vi "Teleop.vi"(10 "Match Info":T1={"Autonomous Elapsed Seconds"=0.0, "TeleOp Elapsed Seconds"=0.0, "Disabled Elapsed Seconds"=0.0, "Visited Autonomous"=FALSE, "Visited TeleOp"=FALSE, "Visited Disabled"=FALSE, "Autonomous Settings"={"Autonomous Style"=enum."Independent", "VI Refnum"=refnum}}, 11 "Call Context":T2) -> ()   [LabVIEW 2018]
doc: "This VI is called for each TeleOp packet received from the DS where the robot is not disabled. It is often used to read from the joysticks and update I/O or to update setpoints for timed control loops. It should complete and return within 20 milliseconds or it may miss DS packets."
uses:
  <vilib>/Rock Robotics/Network Tables/NT Write Numeric Array.vi
  <vilib>/Rock Robotics/Network Tables/NT Read Boolean.vi
  <vilib>/Rock Robotics/Network Tables/NT Write Boolean Array.vi
  <vilib>/Rock Robotics/Network Tables/NT Read Number.vi
  <vilib>/Rock Robotics/Network Tables/NT Write Number.vi
  <vilib>/Rock Robotics/WPI/DriverStation/WPI_DriverStationMatch Info.ctl
  <vilib>/Rock Robotics/WPI/DriverStation/WPI_DriverStationDerivedRobotMode.ctl
panel:
  out "Color":u32(colorbox)
  out "Measured Color":cluster{"R":dbl, "G":dbl, "B":dbl}
  out "Sample Slider 0":dbl(slide) scale=0.0..5.0
  out "Sample Boolean 1":bool
  out "Sample Boolean 0":bool
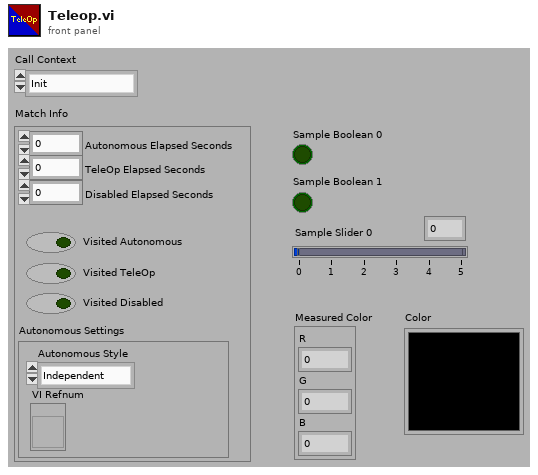
[diagram p1: front panel]
types:
  T1 = typedef "WPI_DriverStationMatch Info.ctl" = cluster{"Autonomous Elapsed Seconds":dbl, "TeleOp Elapsed Seconds":dbl, "Disabled Elapsed Seconds":dbl, "Visited Autonomous":bool, "Visited TeleOp":bool, "Visited Disabled":bool, "Autonomous Settings":cluster{"Autonomous Style":enum16{"Iterative", "Independent"}, "VI Refnum":refnum<vi>}}
  T2 = typedef "WPI_DriverStationDerivedRobotMode.ctl" = enum16{"Init", "Execute", "Stop"}
  T3 = typedef "WPI_RobotDriveDevRef.ctl" = cluster{"DevStatus":errorcluster, "Motors[]":T4[], "Square Inputs":bool, "Max Output":dbl}
  T4 = typedef "WPI_MotorControlDeviceRef.ctl" = cluster{"DeviceStatus":errorcluster, "Type":T5, "PWM":cluster{"PWM Channel":T6, "DeadBand":T7}, "CAN":cluster{"Device Number":u8, "SetOutput VI Ref":variant, "GetOutput VI Ref":variant, "Enable VI Ref":variant, "Disable VI Ref":variant, "Data":variant}, "Invert":bool, "DIO PWM":cluster{"PWM \"Enable\" Channel":T6, "DIOChannel":T8, "PWM Rate":dbl}}
  T5 = typedef "WPI_MotorControlType.ctl" = enum16{"PWM", "CAN", "DIO PWM"}
  T6 = typedef "FPGA_DIOPWMChannel.ctl" = enum8{"PWM 0", "PWM 1", "PWM 2", "PWM 3", "PWM 4", "PWM 5", "PWM 6", "PWM 7", "PWM 8", "PWM 9", "PWM MXP 0", "PWM MXP 1", "PWM MXP 2", "PWM MXP 3", "PWM MXP 4", "PWM MXP 5", "PWM MXP 6", "PWM MXP 7", "PWM MXP 8", "PWM MXP 9", "Invalid"}
  T7 = typedef "WPI_PWMDeadband.ctl" = cluster{"Name":string, "maxPositivePwm":i32, "minPositivePwm":i32, "centerPwm":i32, "maxNegativePwm":i32, "minNegativePwm":i32, "angularRange":u16}
  T8 = typedef "FPGA_DIOChannel.ctl" = enum8{"DIO 0", "DIO 1", "DIO 2", "DIO 3", "DIO 4", "DIO 5", "DIO 6", "DIO 7", "DIO 8", "DIO 9", "DIO MXP 0", "DIO MXP 1", "DIO MXP 2", "DIO MXP 3", "DIO MXP 4", "DIO MXP 5", "DIO MXP 6", "DIO MXP 7", "DIO MXP 8", "DIO MXP 9", "DIO MXP 10", "DIO MXP 11", "DIO MXP 12", "DIO MXP 13", "DIO MXP 14", "DIO MXP 15", "SPI Port CS1", "SPI Port CS2", "SPI Port CS3", "SPI Port MISO", "SPI Port MOSI", "Invalid"}
  T9 = typedef "WPI_JoystickDevRef.ctl" = cluster{"Device":T10}
  T10 = typedef "WPI_JoystickDeviceEnum.ctl" = enum16{"USB 0", "USB 1", "USB 2", "USB 3", "USB 4", "USB 5"}
  T11 = typedef "Color Sensor V3 DevRef.ctl" = cluster{"I2CDevRef":T12}
  T12 = typedef "WPI_I2CDevRef.ctl" = cluster{"DevStatus":errorcluster, "Device Address":u8, "Handle":i32, "I2C Bus":T13}
  T13 = typedef "i2c_bus.ctl" = enum16{"I2C On-Board", "I2C MXP", "Invalid"}
  T14 = typedef "WPI_GyroDevRef.ctl" = cluster{"DevStatus":errorcluster, "Analog Channel":T15, "Gain (VoltsPerDegree/Second)":dbl, "Gyro Type":enum16{"Analog", "XRS450"}, "Handle":i32, "SPI Bus":T16, "Device Found":bool, "Sample Rate":dbl, "Calibrate On Open":bool, "Offset":dbl}
  T15 = typedef "FPGA_AIChannel.ctl" = enum8{"AI 0", "AI 1", "AI 2", "AI 3", "AI MXP 0", "AI MXP 1", "AI MXP 2", "AI MXP 3", "Invalid"}
  T16 = typedef "spi_bus.ctl" = enum16{"SPI On-Board, CS0", "SPI On-Board, CS1", "SPI On-Board, CS2", "SPI On-Board, CS3", "SPI MXP", "Invalid"}
  T17 = typedef "WPI_CompressorDevRef.ctl" = cluster{"DevStatus":errorcluster, "Pneumatics Control Module":u8}
  T18 = typedef "WPI_EncoderDevRef.ctl" = cluster{"DevStatus":errorcluster, "EncoderIndex":T19, "CounterIndex":T20, "DistancePerCount":dbl, "Decoding Type":T21}
  T19 = typedef "FPGA_EncoderIdx.ctl" = enum8{"Enc 0", "Enc 1", "Enc 2", "Enc 3", "Enc 4", "Enc 5", "Enc 6", "Enc 7", "Invalid"}
  T20 = typedef "FPGA_CounterCtrSystemIndex.ctl" = enum8{"Ctr 0", "Ctr 1", "Ctr 2", "Ctr 3", "Ctr 4", "Ctr 5", "Ctr 6", "Ctr 7", "Invalid"}
  T21 = typedef "WPI_EncoderType.ctl" = enum16{"1x", "2x", "4x"}
  T22 = typedef "WPI_AnalogChannelDevRef.ctl" = cluster{"DevStatus":errorcluster, "Analog Channel":T15}
  T23 = typedef "WPI_AccelerometerDevRef.ctl" = cluster{"DevStatus":errorcluster, "Scaling":T24, "Analog Channels":T25, "I2C Bus":T13, "SPI Bus":T16, "Accel Range":T26, "ADXL Axes":T27, "Handle":i32, "Device Address":u8, "Accel Type":enum16{"Analog", "ADXL345 I2C", "ADXL345 SPI", "Internal", "ADXL362 SPI"}}
  T24 = typedef "WPI_AccelerometerScaling.ctl" = cluster{"Gain (VoltsPerG)":dbl, "Center Voltage":dbl}
  T25 = typedef "WPI_AccelerometerAnalogChannels.ctl" = cluster{"X-Axis":T15, "Y-Axis":T15, "Z-Axis":T15}
  T26 = typedef "ADXL345 Range.ctl" = u8
  T27 = typedef "WPI_AccelerometerADXL345 Axes.ctl" = cluster{"X-Axis":bool, "Y-Axis":bool, "Z-Axis":bool}
  T28 = cluster{"X-Axis":dbl, "Y-Axis":dbl, "Z-Axis":dbl}
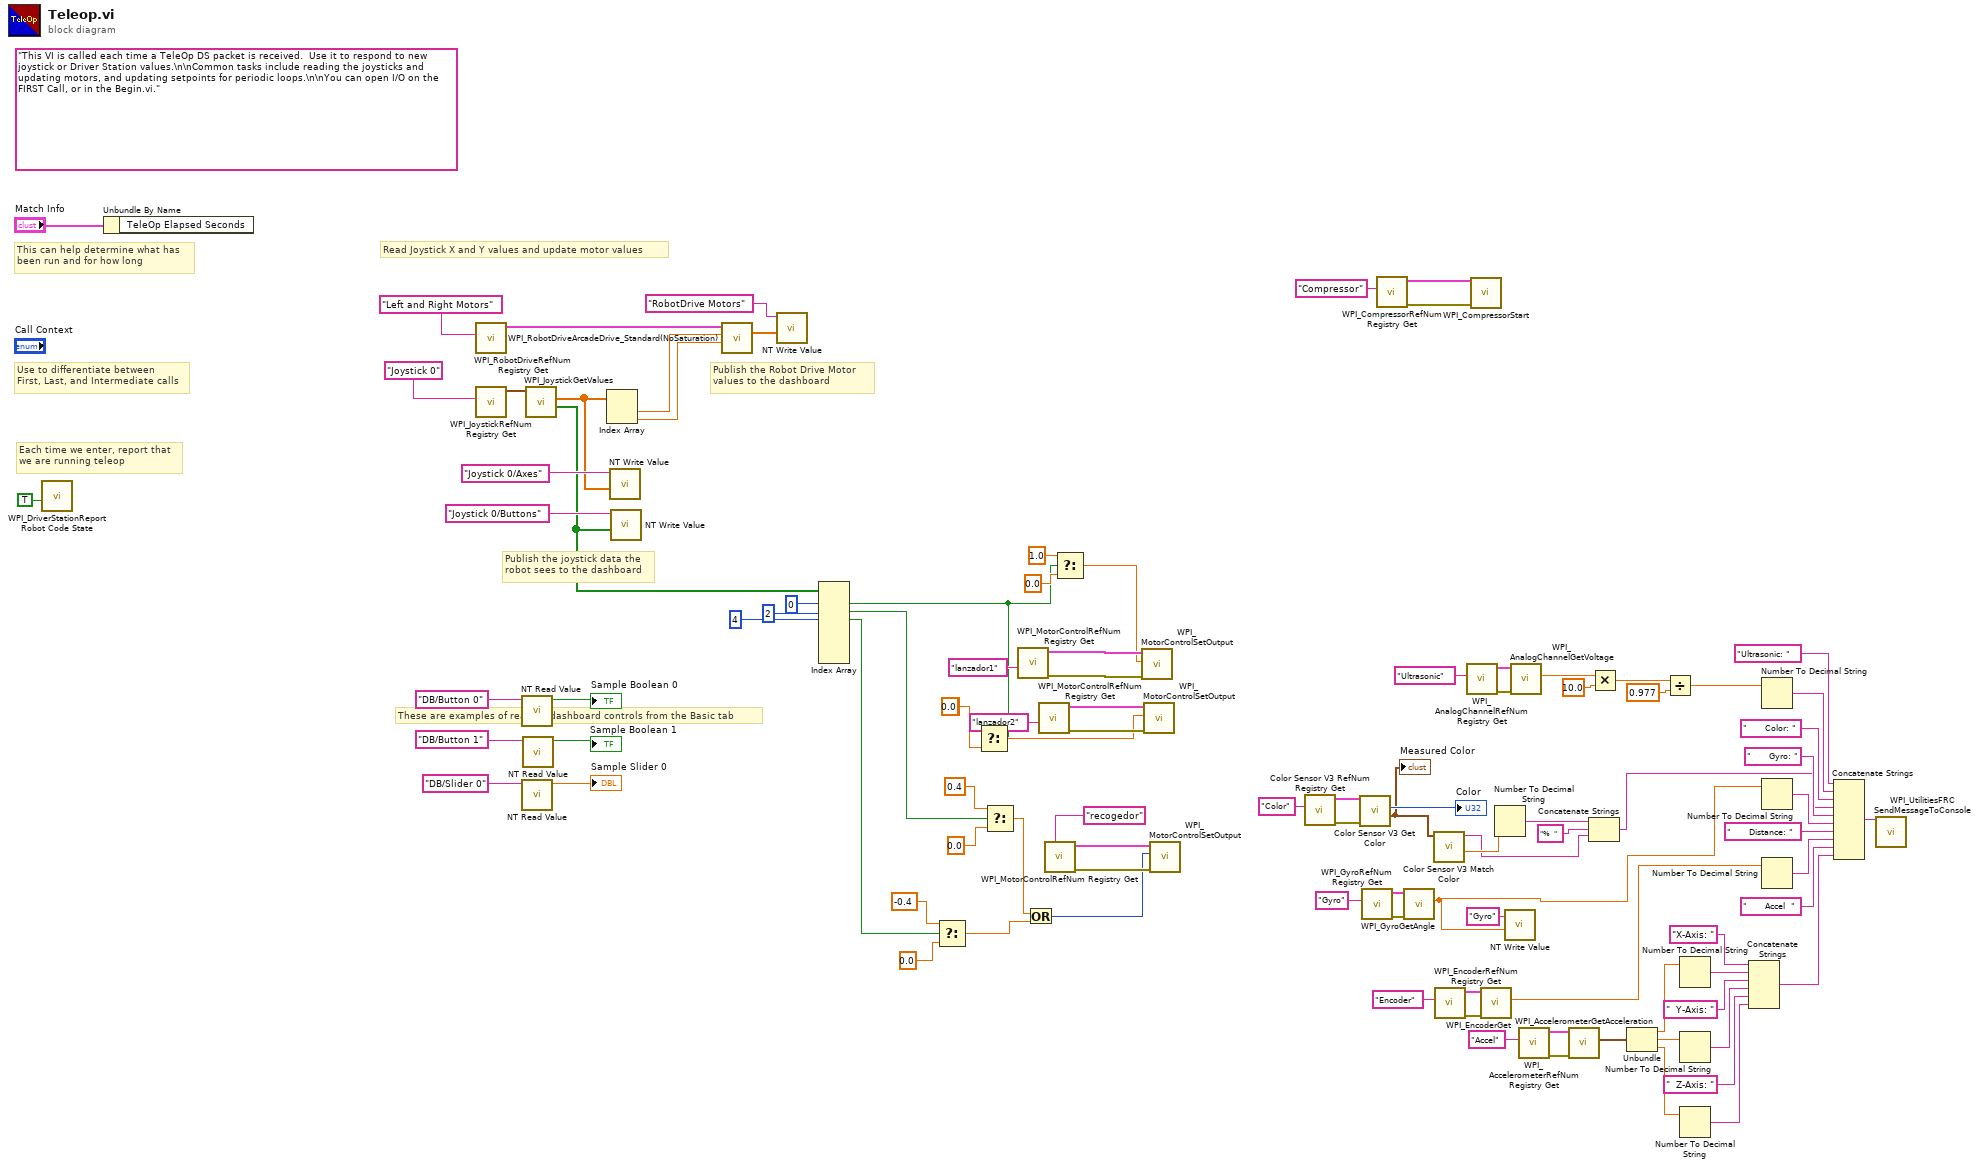
[diagram p0: block diagram]
diagram:
  (unwired) "This VI is called each time a TeleOp DS packet is received.  Use it to respond to new joystick or Driver Station values.\n\nCommon tasks include reading the joysticks and updating motors, and updating setpoints for periodic loops.\n\nYou can open I/O on the FIRST Call, or in the Begin.vi."
  # "These are examples of reading dashboard controls from the Basic tab"
  # "Publish the Robot Drive Motor\nvalues to the dashboard"
  # "Publish the joystick data the\nrobot sees to the dashboard"
  # "Each time we enter, report that\nwe are running teleop"
  # "Use to differentiate between\nFirst, Last, and Intermediate calls"
  # "This can help determine what has\nbeen run and for how long"
  # "Read Joystick X and Y values and update motor values"
  n1 = call <vilib>:"WPI_DriverStationReport Robot Code State.vi"("TeleOp"=TRUE ("Autonomous")) -> ()  [unwired: 10 in, 1 out]
  n2 = Unbundle By Name("Match Info") -> ()  [unwired: 1 out]
  n3 = call <vilib>:"WPI_RobotDriveRefNum Registry Get.vi"("refnum name"="Left and Right Motors") -> ("RobotDriveDevRef"=w99:T3)  [unwired: 1 in, 9 out]
  n4 = call <vilib>:"WPI_JoystickRefNum Registry Get.vi"("refnum name"="Joystick 0") -> ("JoystickDevRef"=w96:T9)  [unwired: 1 in, 9 out]
  n5 = call-poly <vilib>:"NT Read Value.vi"("Name"="DB/Button 0" ("refnum name")) -> ("Boolean"=→"Sample Boolean 0":bool)  [unwired: 9 in, 1 out]
  n6 = call-poly <vilib>:"NT Read Value.vi"("Name"="DB/Slider 0" ("refnum name")) -> ("Numeric"=→"Sample Slider 0":dbl)  [unwired: 9 in, 1 out]
  n7 = call-poly <vilib>:"NT Read Value.vi"("Name"="DB/Button 1" ("refnum name")) -> ("Boolean"=→"Sample Boolean 1":bool)  [unwired: 9 in, 1 out]
  n8 = call <vilib>:"WPI_JoystickGetValues.vi"("JoystickDevRef"=w96) -> ("Buttons"=w82:bool[], "Axes"=w91:dbl[])  [unwired: 6 in, 3 out]
  n9 = Index Array(array=w91) -> (element #1=w98:dbl, element #2=w94:dbl)  [unwired: 2 in]
  n10 = call-poly <vilib>:"NT Write Value.vi"("Numeric Array"=w91, "Name"="Joystick 0/Axes") -> ()  [unwired: 9 in, 1 out]
  n11 = call-poly <vilib>:"NT Write Value.vi"("Boolean Array"=w82, "Name"="Joystick 0/Buttons") -> ()  [unwired: 9 in, 1 out]
  n12 = call <vilib>:"WPI_RobotDriveArcadeDrive_Standard(NoSaturation).vi"("Y axis value"=w94, "X axis value"=w98, "RobotDriveDevRef"=w99) -> ("Motor Values"=w84:dbl[])  [unwired: 1 in, 7 out]
  n13 = call-poly <vilib>:"NT Write Value.vi"("Numeric Array"=w84, "Name"="RobotDrive Motors") -> ()  [unwired: 9 in, 1 out]
  n14 = Index Array(array=w82, index #1=0 ("index"), index #2=2 ("index"), index #3=4 ("index")) -> (element #1=w62:bool, element #2=w58:bool, element #3=w54:bool)  [unwired: 5 in, 5 out]
  n15 = Select(t=-0.4, s=w54, f=0.0) -> (s? t:f=w57:dbl)
  n16 = Select(t=1.0, s=w62, f=0.0) -> (s? t:f=w70:dbl)
  n17 = Select(t=0.4, s=w58, f=0.0) -> (s? t:f=w61:dbl)
  n18 = call <vilib>:"WPI_MotorControlRefNum Registry Get.vi"("refnum name"="lanzador1") -> ("error out"=w78:errorcluster, "MotorControlDevRef"=w79:T4)  [unwired: 9 in]
  n19 = Or(x=w61, y=w57) -> (x .or. y?=w56:i32)
  n20 = call <vilib>:"WPI_MotorControlRefNum Registry Get.vi"("refnum name"="lanzador2") -> ("error out"=w72:errorcluster, "MotorControlDevRef"=w73:T4)  [unwired: 9 in]
  n21 = call <vilib>:"WPI_MotorControlRefNum Registry Get.vi"("refnum name"="recogedor") -> ("error out"=w66:errorcluster, "MotorControlDevRef"=w67:T4)  [unwired: 9 in]
  n22 = Select(t=1.0, s=w62, f=0.0) -> (s? t:f=w76:dbl)
  n23 = call <vilib>:"WPI_MotorControlSetOutput.vi"("error in (no error)"=w78, "Output"=w76, "MotorControlDevRef"=w79) -> ()  [unwired: 6 in, 3 out]
  n24 = call <vilib>:"WPI_MotorControlSetOutput.vi"("error in (no error)"=w72, "Output"=w70, "MotorControlDevRef"=w73) -> ()  [unwired: 6 in, 3 out]
  n25 = call <vilib>:"WPI_MotorControlSetOutput.vi"("error in (no error)"=w66, "Output"=w56, "MotorControlDevRef"=w67) -> ()  [unwired: 6 in, 3 out]
  n26 = call <vilib>:"Color Sensor V3 RefNum Registry Get.vi"("refnum name"="Color") -> ("error out"=w12:errorcluster, "ColorSensorDevRef"=w13:T11)  [unwired: 9 in]
  n27 = call <vilib>:"Color Sensor V3 Get Color.vi"("error in (no error)"=w12, "ColorSensorDevRef"=w13) -> ("Normalized Color"=w9:cluster{"R":dbl, "G":dbl, "B":dbl}, "Color"=→"Color":u32)  [unwired: 6 in, 2 out]
  "Measured Color" <- w9
  n28 = call <vilib>:"WPI_GyroRefNum Registry Get.vi"("refnum name"="Gyro") -> ("error out"=w40:errorcluster, "GyroDevRef"=w41:T14)  [unwired: 9 in]
  n29 = call <vilib>:"WPI_CompressorRefNum Registry Get.vi"("refnum name"="Compressor") -> ("error out"=w2:errorcluster, "CompressorDevRef"=w3:T17)  [unwired: 9 in]
  n30 = call <vilib>:"WPI_GyroGetAngle.vi"("error in"=w40, "GyroDevRef"=w41) -> ("Angle"=w14:dbl)  [unwired: 5 in, 4 out]
  n31 = call <vilib>:"Color Sensor V3 Match Color.vi"("Measured Color"=w9) -> ("Confidence"=w8:dbl, "Matched Color Name"=w5:string)  [unwired: 8 in, 1 out]
  n32 = call <vilib>:"WPI_EncoderRefNum Registry Get.vi"("refnum name"="Encoder") -> ("error out"=w35:errorcluster, "EncoderDevRef"=w36:T18)  [unwired: 9 in]
  n33 = call <vilib>:"WPI_AnalogChannelRefNum Registry Get.vi"("refnum name"="Ultrasonic") -> ("error out"=w52:errorcluster, "AIDeviceRef"=w53:T22)  [unwired: 9 in]
  n34 = call <vilib>:"WPI_CompressorStart.vi"("error in (no error)"=w2, "CompressorDevRef"=w3) -> ()  [unwired: 8 in, 2 out]
  n35 = call <vilib>:"WPI_EncoderGet.vi"("error in (no error)"=w35, "EncoderDevRef"=w36) -> ("Distance"=w33:dbl)  [unwired: 4 in, 5 out]
  n36 = Number To Decimal String(number=w8) -> (decimal integer string=w7:string)  [unwired: 1 in]
  n37 = call-poly <vilib>:"NT Write Value.vi"("Numeric"=w14, "Name"="Gyro") -> ()  [unwired: 9 in, 1 out]
  n38 = call <vilib>:"WPI_AnalogChannelGetVoltage.vi"("error in (no error)"=w52, "AIDeviceRef"=w53) -> ("Voltage"=w50:dbl)  [unwired: 7 in, 2 out]
  n39 = call <vilib>:"WPI_AccelerometerRefNum Registry Get.vi"("refnum name"="Accel") -> ("error out"=w28:errorcluster, "AccelerometerDevRef"=w29:T23)  [unwired: 9 in]
  n40 = call <vilib>:"WPI_AccelerometerGetAcceleration.vi"("error in"=w28, "AccelerometerDevRef"=w29) -> ("Accelerations"=w27:T28)  [unwired: 7 in, 2 out]
  n41 = Concatenate Strings(w7, "%  " ("string"), w5) -> (w4:string)
  n42 = Multiply(x=w50, y=10.0) -> (x*y=w48:dbl)
  n43 = Unbundle(w27) -> ("X-Axis"=w24:dbl, "Y-Axis"=w22:dbl, "Z-Axis"=w21:dbl)
  n44 = Divide(x=w48, y=0.977) -> (x/y=w46:dbl)
  n45 = Number To Decimal String(number=w24) -> (decimal integer string=w23:string)  [unwired: 1 in]
  n46 = Number To Decimal String(number=w22) -> (decimal integer string=w20:string)  [unwired: 1 in]
  n47 = Number To Decimal String(number=w21) -> (decimal integer string=w19:string)  [unwired: 1 in]
  n48 = Concatenate Strings("X-Axis: " ("string"), w23, "  Y-Axis: " ("string"), w20, "  Z-Axis: " ("string"), w19) -> (w16:string)
  n49 = Number To Decimal String(number=w46) -> (decimal integer string=w44:string)  [unwired: 1 in]
  n50 = Number To Decimal String(number=w14) -> (decimal integer string=w38:string)  [unwired: 1 in]
  n51 = Number To Decimal String(number=w33) -> (decimal integer string=w31:string)  [unwired: 1 in]
  n52 = Concatenate Strings("Ultrasonic: " ("string"), w44, "      Color: " ("string"), w4, "      Gyro: " ("string"), w38, "      Distance: " ("string"), w31, "      Accel  " ("string"), w16) -> (w37:string)
  n53 = call <vilib>:"WPI_UtilitiesFRC SendMessageToConsole.vi"("Message"=w37) -> ()  [unwired: 14 in, 1 out]
